vi "iow56_i2c_read.vi"() -> ()   [LabVIEW 2011]
uses:
  IOWarrior V150.llb/IOWarrior_Type.ctl
panel:
  out "ACK Result":i32[](array[numeric]) format="%.0x"
  out "Error":errorcluster caption="error"
  out "Read Result":i32[](array[numeric]) format="%.0x"
  in  "?":u8 format="%x"
  out "type of Warrior":T1
  # "I2C-Address"
  # "Bytes to Read"
  # "Error Messages"
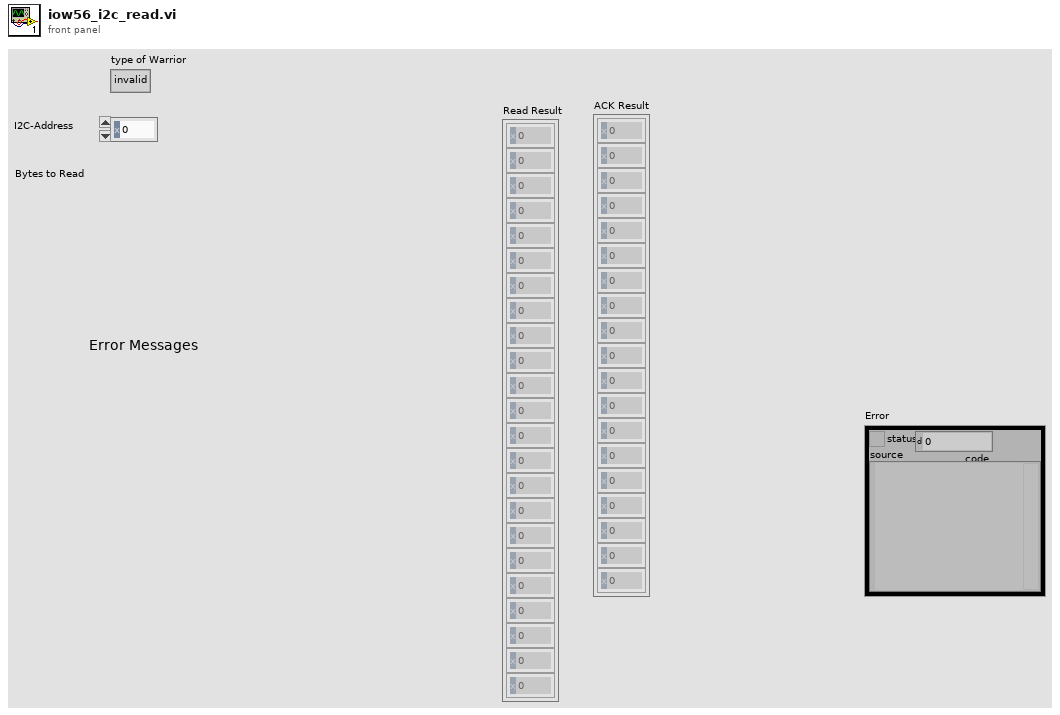
[diagram p1: front panel]
types:
  T1 = typedef "IOWarrior_Type.ctl" = enum16{"invalid", "IOW24", "IOW40", "IOW56", "IOPV1", "IOPV2", "IOW28"}
  T2 = typedef "IOWarrior_Handle.ctl" = cluster{"Handle":u32, "Serial Number":string, "type of Warrior":T1, "Root Handle":bool, "Revision":u16}
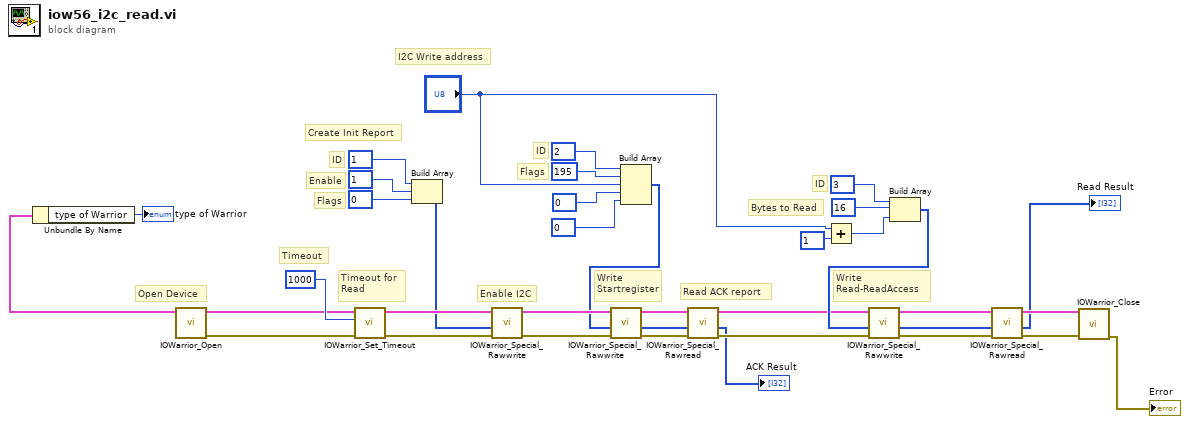
[diagram p0: block diagram]
diagram:
  # "Read ACK report"
  # "Flags"
  # "ID"
  # "Write\nStartregister"
  # "Write \nRead-ReadAccess"
  # "ID"
  # "Bytes to Read"
  # "I2C Write address"
  # "Create Init Report"
  # "Flags"
  # "Enable"
  # "ID"
  # "Timeout"
  # "Open Device"
  # "Enable I2C"
  # "Timeout for\nRead"
  n1 = call "IOWarrior_Open.vi"() -> ("err out"=w33:errorcluster, "IOWarriorHandle"=w31:T2)  [unwired: 9 in, 1 out]
  n2 = Unbundle By Name(w31) -> ("type of Warrior"=→"type of Warrior":T1)
  n3 = call "IOWarrior_Set_Timeout.vi"("err in"=w33, "timeout_ms(1000)"=1000, "devHandle"=w31) -> ("err out"=w36:errorcluster, "devHandleout"=w35:T2)  [unwired: 6 in, 1 out]
  n4 = Build Array(u8 1, u8 1, u8 0) -> (w27:u8[])
  n5 = call "IOWarrior_Special_Rawwrite.vi"("err in"=w36, "Array_in"=w27, "devHandle"=w35) -> ("err out"=w22:errorcluster, "devHandleout"=w21:T2)  [unwired: 6 in, 1 out]
  n6 = Build Array(u8 2, u8 195, "?", u8 0, u8 0) -> (w19:u8[])
  n7 = call "IOWarrior_Special_Rawwrite.vi"("err in"=w22, "Array_in"=w19, "devHandle"=w21) -> ("err out"=w14:errorcluster, "array_out"=w12:u8[], "devHandleout"=w16:T2)  [unwired: 6 in]
  n8 = call "IOWarrior_Special_Rawread.vi"("err in"=w14, "array"=w12, "devHandle"=w16) -> ("err out"=w13:errorcluster, "arrayout"=→"ACK Result":u8[], "devHandleout"=w15:T2)  [unwired: 6 in]
  n9 = Add(x="?", y=u8 1) -> (x+y=w17:u8)
  n10 = Build Array(u8 3, u8 16, w17) -> (w18:u8[])
  n11 = call "IOWarrior_Special_Rawwrite.vi"("err in"=w13, "Array_in"=w18, "devHandle"=w15) -> ("err out"=w10:errorcluster, "array_out"=w9:u8[], "devHandleout"=w11:T2)  [unwired: 6 in]
  n12 = call "IOWarrior_Special_Rawread.vi"("err in"=w10, "array"=w9, "devHandle"=w11) -> ("err out"=w7:errorcluster, "arrayout"=→"Read Result":u8[], "devHandleout"=w6:T2)  [unwired: 6 in]
  n13 = call "IOWarrior_Close.vi"("err in"=w7, "devHandle"=w6) -> ("err out"=→"Error":errorcluster)  [unwired: 8 in, 1 out]
